vi "Double pipeline.vi"(8 "input valid":bool, 11 "data in":T1[](array[typedef])=[{"I"=0.0, "Q"=0.0, "overflow"=FALSE}, {"I"=0.0, "Q"=0.0, "overflow"=FALSE}, {"I"=0.0, "Q"=0.0, "overflow"=FALSE}, {"I"=0.0, "Q"=0.0, "overflow"=FALSE}]) -> (0 "input valid pipe":bool, 3 "data in pipe":T1[](array[typedef]))   [LabVIEW 2025]
uses:
  <instrlib>/_niInstr/DSP/v1/Shared/Public/IQ Data.ctl
  <instrlib>/_niInstr/DSP Control/Common/v2/FPGA/niInstr DSP Control Common v2 FPGA.lvlib
  <instrlib>/_niInstr/DSP/v1/Shared/niInstr DSP v1 Shared.lvlib
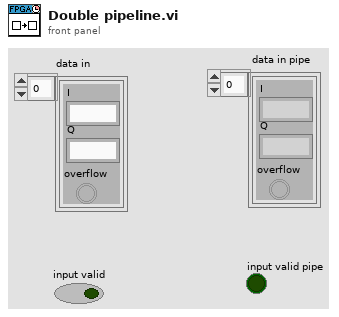
[diagram p1: front panel]
types:
  T1 = typedef "niInstr DSP v1 Shared.lvlib/IQ Data.ctl" = cluster{"I":fxp<+/-,18,1>, "Q":fxp<+/-,18,1>, "overflow":bool}
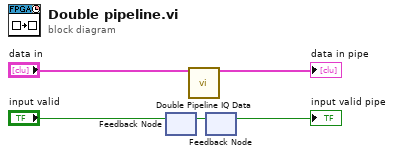
[diagram p0: block diagram]
diagram:
  n1 = feedback #1() -> (w1:bool)  [unwired: 1 in]
  n2 = feedback-in #1("input valid") -> ()
  n3 = call <instrlib>:"Double Pipeline IQ Data.vi"("data in"="data in") -> ("data out"=→"data in pipe":T1[])  [unwired: 14 in]
  n4 = feedback #2() -> (→"input valid pipe":bool)  [unwired: 1 in]
  n5 = feedback-in #2(w1) -> ()
